vi "Main.vi"(11 "Module Admin":refnum<class "Delacor_lib_QMH_Cloneable Module Admin.lvclass">) -> ()   [LabVIEW 2024, in "ClonSubpanel.lvlib"]
doc: "This template is based off of the Queued Message Handler design pattern and the Queued Message Handler project template that ships with LabVIEW.\n\nThe main difference is that the queue is private to this module and communication between modules is performed via Broadcast and Request events.\n\nRequest events are wrapped in public API methods and are handled in the Event Handling Loop (EHL) of this VI. Any module can register for Broadcast events sent by this module. The EHL generates messages based on user interface actions.\n\nThe Message Handling Loop (MHL) processes messages generated by the EHL, or by other messages. The messages are string values, so new messages can be added easily to the Message Cases case structure in the MHL. Each message cluster can also provide an optional value for Message Data, which is a variant that can be converted to whatever message-specific data is required.\n_____\nBased on DQMH Dev Tools: Project Template 7.1.0.1503."
uses:
  ClonSubpanel.lvlib
  <vilib>/Delacor/Delacor QMH/Libraries/Cloneable Module Admin_class/Delacor_lib_QMH_Cloneable Module Admin.lvclass
  C:/Program Files (x86)/National Instruments/LabVIEW 2024/vi.lib/Delacor/Delacor QMH/Libraries/Module Admin_class/Delacor_lib_QMH_Module Admin.lvclass
  Module Data--cluster.ctl
  <vilib>/Delacor/Delacor QMH/Libraries/Message Queue_class/Delacor_lib_QMH_Message Queue.lvclass/Delacor_lib_QMH_Message Queue.ctl
  <vilib>/Delacor/Delacor QMH/Libraries/Cloneable Module Admin_class/Delacor_lib_QMH_Cloneable Module Admin.lvclass/Delacor_lib_QMH_Cloneable Module Admin.ctl
  Stop Argument--cluster.ctl
  <vilib>/Delacor/Delacor QMH/Libraries/Module Admin_class/Delacor_lib_QMH_Module Admin.lvclass/Delacor_lib_QMH_Module Admin.ctl
  Draw FP in Supbpanel Argument--cluster.ctl
  Remove FP from Subpanel Argument--cluster.ctl
  <vilib>/Utility/miscctls.llb/LVPointTypeDef.ctl
  <vilib>/Delacor/Delacor QMH/Libraries/Message Queue_class/Delacor_lib_QMH_Enqueue Message (Single).vi
  <vilib>/Delacor/Delacor QMH/Libraries/Cloneable Module Admin_class/Delacor_lib_QMH_Get Module ID.vi
  <vilib>/Delacor/Delacor QMH/Libraries/Module Admin_class/Delacor_lib_QMH_Get External Launch.vi
  <vilib>/Delacor/Delacor QMH/Libraries/Message Queue_class/Delacor_lib_QMH_Message Queue.lvclass
panel:
  out "error out":errorcluster
  out "Status":string
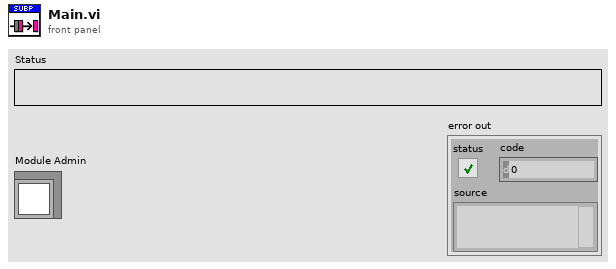
[diagram p1: front panel]
types:
  T1 = typedef "ClonSubpanel.lvlib/Request Events--cluster.ctl" = cluster{"Stop Module":refnum<user-event>, "Show Panel":refnum<user-event>, "Hide Panel":refnum<user-event>, "Show Diagram":refnum<user-event>, "Get Module Execution Status":refnum<user-event>, "Draw FP in Supbpanel":refnum<user-event>, "Remove FP from Subpanel":refnum<user-event>}
  T2 = typedef "ClonSubpanel.lvlib/Module Data--cluster.ctl" = cluster{"Status":string, "Sub Panel":refnum<vi>}
  T3 = enum32{"invalid lock state", "Not Locked", "Locked (No Password)", "Password-protected"}
  T4 = typedef "ClonSubpanel.lvlib/Stop Argument--cluster.ctl" = cluster{"Module ID":i32, "Origin":string, "Exit via Stop Module Req?":bool, "Wait for Module to stop?":bool}
  T5 = typedef "ClonSubpanel.lvlib/Draw FP in Supbpanel Argument--cluster.ctl" = cluster{"Module ID":i32, "Sub Panel":refnum<vi>}
  T6 = typedef "ClonSubpanel.lvlib/Remove FP from Subpanel Argument--cluster.ctl" = cluster{"Module ID":i32, "Boolean":bool}
  T7 = typedef "LVPointTypeDef.ctl" = cluster{"Horizontal":i16, "Vertical":i16}
  T8 = enum32{"Invalid", "Standard", "Closed", "Hidden", "Minimized", "Maximized"}
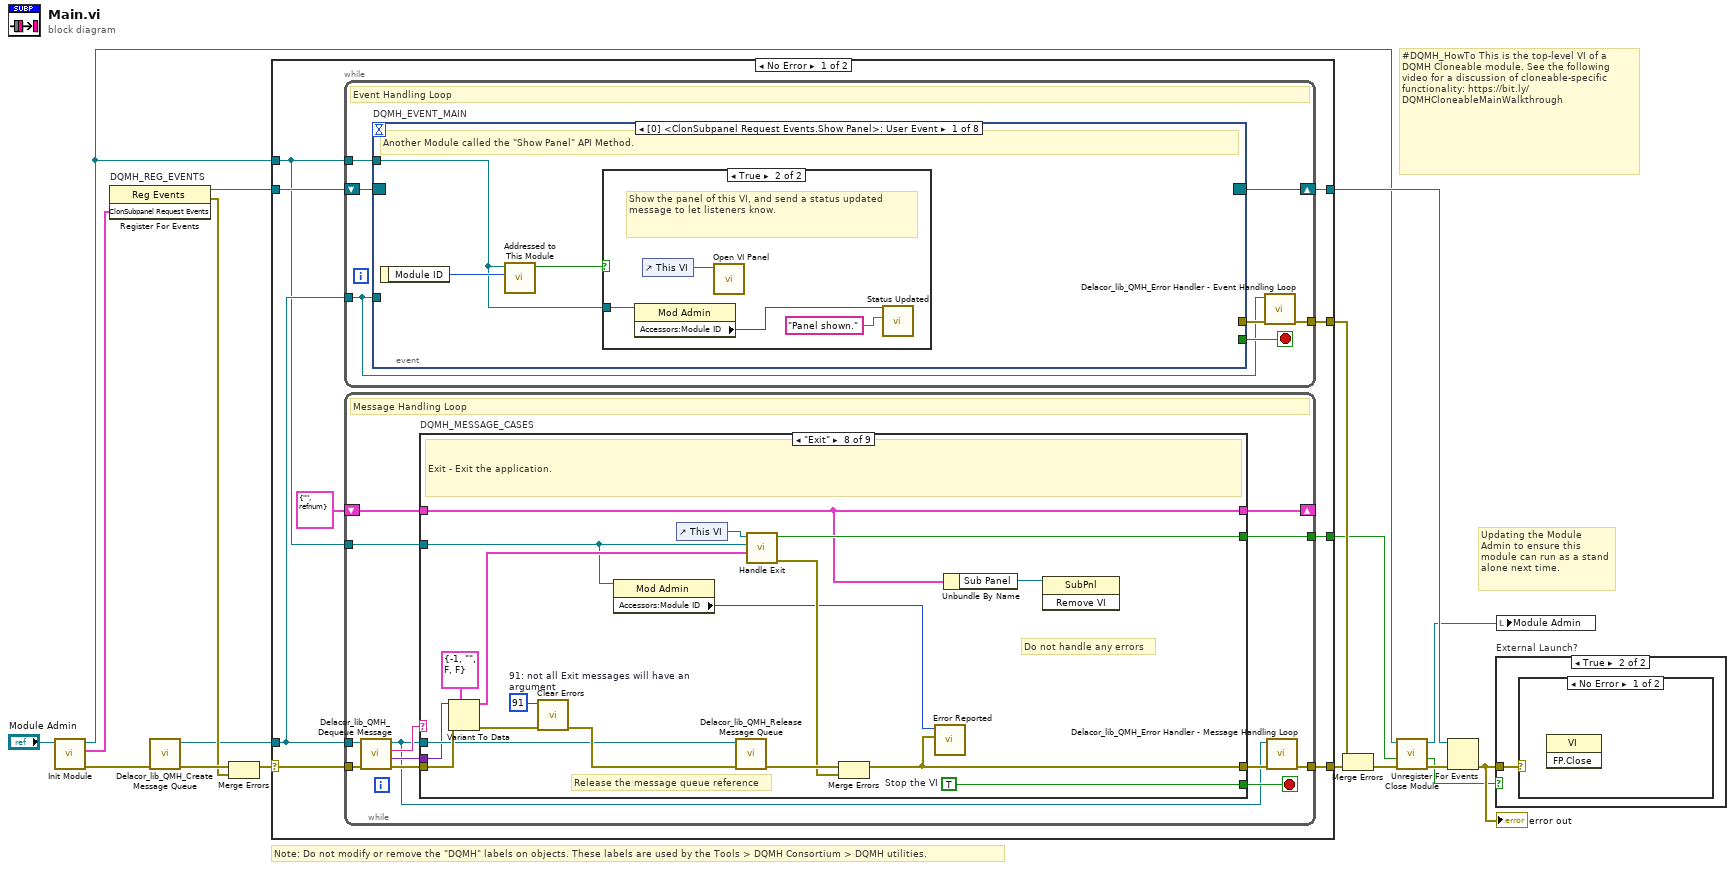
[diagram p0: block diagram]
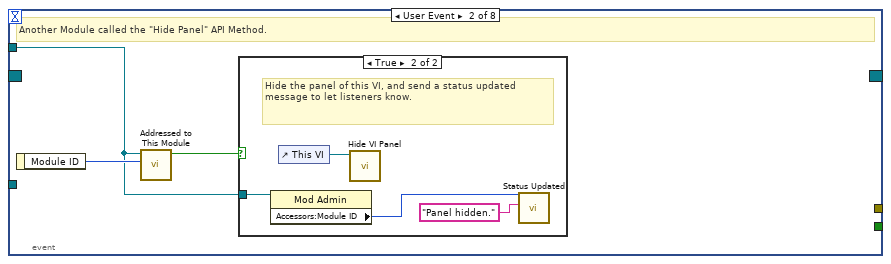
[diagram p3: hidden frame]
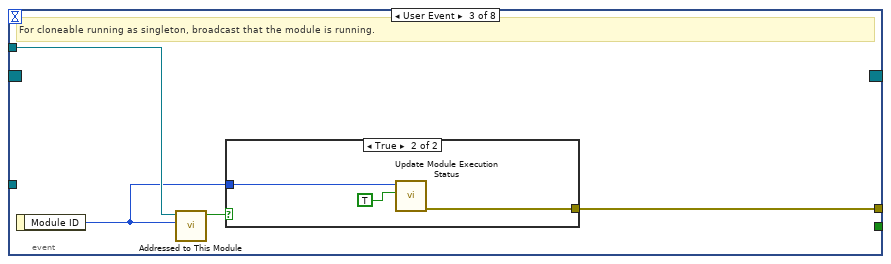
[diagram p5: hidden frame]
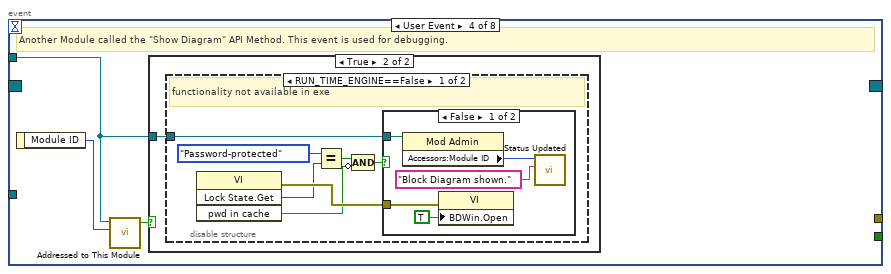
[diagram p7: hidden frame]
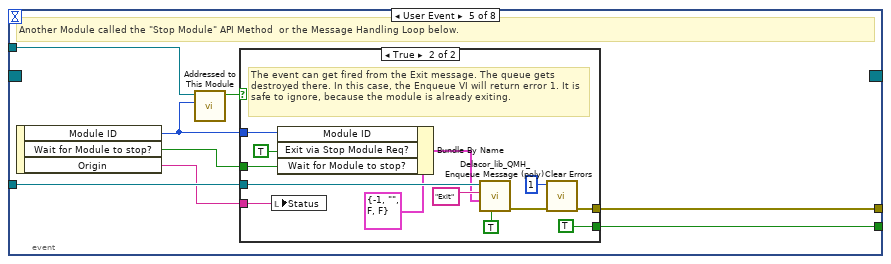
[diagram p11: hidden frame]
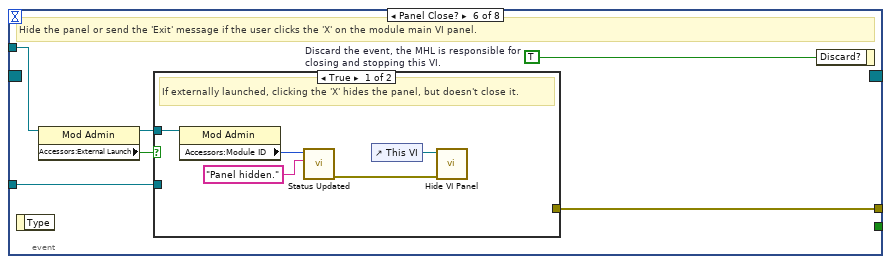
[diagram p13: hidden frame]
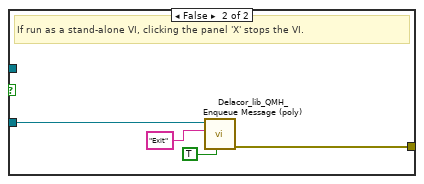
[diagram p14: hidden frame]
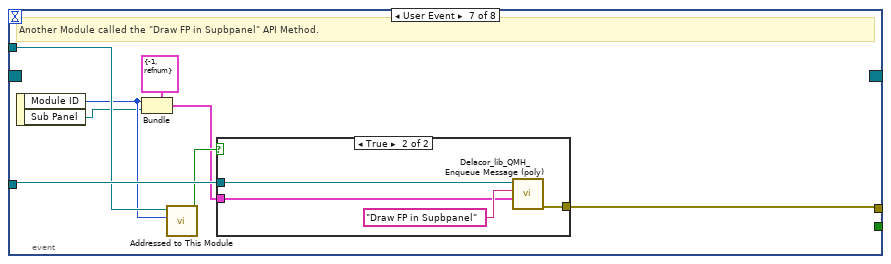
[diagram p15: hidden frame]
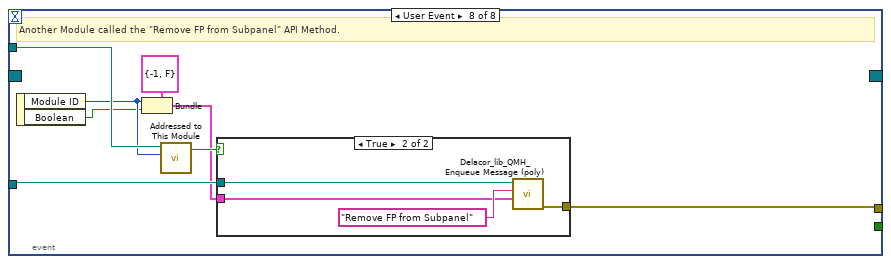
[diagram p17: hidden frame]
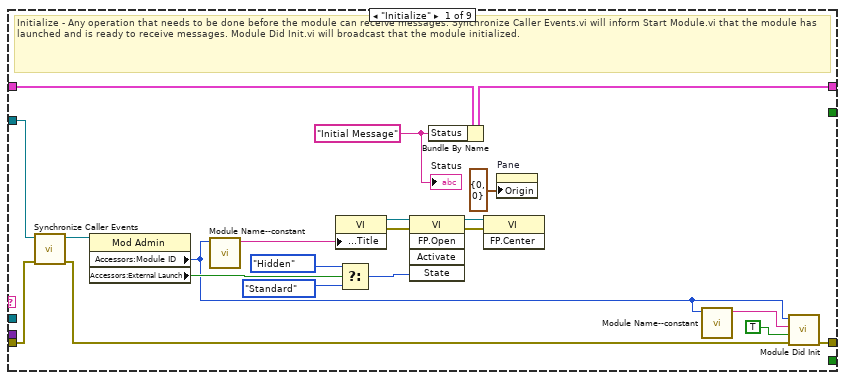
[diagram p19: hidden frame]
diagram:
  # "#DQMH_HowTo This is the top-level VI of a DQMH Cloneable module. See the following video for a discussion of cloneable-specific functionality: https://bit.ly/DQMHCloneableMainWalkthrough"
  # "Note: Do not modify or remove the \"DQMH\" labels on objects. These labels are used by the Tools > DQMH Consortium > DQMH utilities."
  # "Updating the Module Admin to ensure this module can run as a stand alone next time."
  n1 = call "Init Module.vi"("Cloneable Module Admin in"="Module Admin") -> ("error out"=w15:errorcluster, "ClonSubpanel Request Events"=w7:T1, "Cloneable Module Admin out"=w4:refnum<class "Delacor_lib_QMH_Cloneable Module Admin.lvclass">)  [unwired: 8 in]
  n2 = register-events "DQMH_REG_EVENTS"(w7) -> (reference out=w8:refnum<event-registration>, error out=w10:errorcluster)  [unwired: 2 in]
  n3 = call <vilib>:"Delacor_lib_QMH_Create Message Queue.vi"("error in"=w15) -> ("error out"=w12:errorcluster, "Message Queue"=w6:refnum<class "Delacor_lib_QMH_Message Queue.lvclass">)  [unwired: 9 in]
  n4 = Merge Errors(w12, w10) -> (w11:errorcluster)
  n5 = case shown="No Error" w11 {
    selector: w11 -> [w25 w267]
    tunnel: [w27 w266] -> w16
    tunnel: [w24 w265] -> w9
    tunnel: w8 -> [w22 w265]
    tunnel: w6 -> [w21 w258]
    tunnel: [w26 _] -> w17
    tunnel: w4 -> [w20 w261]
    tunnel: [w19 _] -> w2
    frame No Error {
      n6 = while {
        tunnel: w21 -> [w28]
        shift-right: [w31] -> w24
        shift-left: w22 -> [w32]
        tunnel: [w33] -> w26
        tunnel: w20 -> [w29]
        stop <- w30 stop-if-true
        # "Event Handling Loop"
        n7 = event "DQMH_EVENT_MAIN" shown="[0] <ClonSubpanel Request Events.Show Panel>: User Event" {
          selector: w32 -> [_ _ _ _ _ _ _ _]
          dyn-events: [_ _ _ _ _ _ _ _] -> w31
          timeout: _ -> [_ _ _ _ _ _ _ _]
          tunnel: [_ _ _ _ w75 _ _ _] -> w30
          tunnel: w28 -> [_ _ _ _ w78 w95 w115 w127]
          tunnel: [_ _ w52 _ w79 w98 w108 w120] -> w34
          tunnel: w29 -> [w35 w42 w50 w56 w77 w96 w113 w125]
          event User Event {
            # "Another Module called the \"Show Panel\" API Method."
            n8 = event-data() -> ("Module ID"=w36:i32)  [unwired: 1 in]
            n9 = call "Addressed to This Module.vi"("Module ID from Argument"=w36, "Module Admin"=w35) -> ("Addressed to this instance?"=w37:bool)  [unwired: 8 in, 1 out]
            n10 = case shown="True" w37 {
              tunnel: w35 -> [_ w39]
              frame False {
              }
              frame True {
                # "Show the panel of this VI, and send a status updated message to let listeners know."
                n11 = property on="Property Node" class="Mod Admin"(reference=w39) -> ("Accessors:Module ID"=w38:i32)  [unwired: 1 in, 2 out]
                n12 = control-ref of="This VI"() -> (w41:refnum<vi>)
                n13 = call "Open VI Panel.vi"("VI"=w41) -> ()  [unwired: 10 in, 1 out]
                n14 = call "Status Updated.vi"("Status"="Panel shown." ("format string"), "Module ID"=w38) -> ()  [unwired: 9 in, 1 out]
              }
            }
          }
          event User Event {
            # "Another Module called the \"Hide Panel\" API Method."
            n15 = event-data() -> ("Module ID"=w43:i32)  [unwired: 1 in]
            n16 = call "Addressed to This Module.vi"("Module ID from Argument"=w43, "Module Admin"=w42) -> ("Addressed to this instance?"=w44:bool)  [unwired: 8 in, 1 out]
            n17 = case shown="True" w44 {
              tunnel: w42 -> [_ w46]
              frame False {
              }
              frame True {
                # "Hide the panel of this VI, and send a status updated message to let listeners know."
                n18 = property on="Property Node" class="Mod Admin"(reference=w46) -> ("Accessors:Module ID"=w45:i32)  [unwired: 1 in, 2 out]
                n19 = control-ref of="This VI"() -> (w48:refnum<vi>)
                n20 = call "Hide VI Panel.vi"("VI"=w48) -> ()  [unwired: 10 in, 1 out]
                n21 = call "Status Updated.vi"("Status"="Panel hidden." ("format string"), "Module ID"=w45) -> ()  [unwired: 9 in, 1 out]
              }
            }
          }
          event User Event {
            # "For cloneable running as singleton, broadcast that the module is running."
            n22 = event-data() -> ("Module ID"=w49:i32)  [unwired: 1 in]
            n23 = call "Addressed to This Module.vi"("Module ID from Argument"=w49, "Module Admin"=w50) -> ("Addressed to this instance?"=w51:bool)  [unwired: 8 in, 1 out]
            n24 = case shown="True" w51 {
              tunnel: [_ w55] -> w52
              tunnel: w49 -> [_ w54]
              frame False {
              }
              frame True {
                n25 = call "Update Module Execution Status.vi"("Running?"=TRUE, "Module ID"=w54) -> ("error out"=w55:errorcluster)  [unwired: 9 in]
              }
            }
          }
          event User Event {
            # "Another Module called the \"Show Diagram\" API Method. This event is used for debugging."
            n26 = event-data() -> ("Module ID"=w57:i32)  [unwired: 1 in]
            n27 = call "Addressed to This Module.vi"("Module ID from Argument"=w57, "Module Admin"=w56) -> ("Addressed to this instance?"=w58:bool)  [unwired: 8 in, 1 out]
            n28 = case shown="True" w58 {
              tunnel: w56 -> [_ w59]
              frame False {
              }
              frame True {
                n29 = disable-structure shown="RUN_TIME_ENGINE==False" {
                  disable-tunnel: w59 -> [w60 _]
                  frame condition #0 (active) {
                    # "functionality not available in exe"
                    n30 = invoke on="Invoke Node" class="VI" method="Lock State.Get"() -> (error out=w66:errorcluster, "Get Lock State"=w65:T3, "pwd in cache"=w62:bool)  [unwired: 4 in, 1 out]
                    n31 = Equal?(x=T3."Password-protected", y=w65) -> (x = y?=w63:bool)
                    n32 = Compound Arithmetic op=AND(w63, invert w62) -> (w61:bool)
                    n33 = case shown="False" w61 {
                      tunnel: w66 -> [w71 _]
                      tunnel: w60 -> [w68 _]
                      frame False {
                        n34 = property on="Property Node" class="Mod Admin"(reference=w68) -> ("Accessors:Module ID"=w67:i32)  [unwired: 1 in, 2 out]
                        n35 = property on="Property Node" class="VI"(error in=w71, "BDWin.Open"=TRUE ("Block Diagram Window:Open")) -> ()  [unwired: 1 in, 2 out]
                        n36 = call "Status Updated.vi"("Status"="Block Diagram shown." ("format string"), "Module ID"=w67) -> ()  [unwired: 9 in, 1 out]
                      }
                      frame True {
                        # "Password-protected VI, and the password is not in the cache. Do not show the diagram."
                      }
                    }
                  }
                  frame condition #1 {
                  }
                }
              }
            }
          }
          event User Event {
            # "Another Module called the \"Stop Module\" API Method  or the Message Handling Loop below."
            n37 = event-data() -> ("Module ID"=w73:i32, "Wait for Module to stop?"=w74:bool, "Origin"=w72:string)  [unwired: 1 in]
            n38 = call "Addressed to This Module.vi"("Module ID from Argument"=w73, "Module Admin"=w77) -> ("Addressed to this instance?"=w76:bool)  [unwired: 8 in, 1 out]
            n39 = case shown="True" w76 {
              tunnel: [_ w91] -> w79
              tunnel: w78 -> [_ w87]
              tunnel: [_ TRUE] -> w75
              tunnel: w74 -> [_ w82]
              tunnel: w73 -> [_ w84]
              tunnel: w72 -> [_ w80]
              frame False {
              }
              frame True {
                # "The event can get fired from the Exit message. The queue gets destroyed there. In this case, the Enqueue VI will return error 1. It is safe to ignore, because the module is already exiting."
                n40 = local write "Status"(w80) -> ()
                n41 = Bundle By Name(cluster=T4 {"Module ID"=-1, "Origin"="", "Exit via Stop Module Req?"=FALSE, "Wait for Module to stop?"=FALSE} ("Stop Argument"), "Module ID"=w84, "Exit via Stop Module Req?"=TRUE, "Wait for Module to stop?"=w82) -> (w81:T4)
                n42 = call-poly <vilib>:"Delacor_lib_QMH_Enqueue Message (poly).vi"("Priority Message? (F)"=TRUE, "Message Data"=w81, "Message"="Exit", "Message Queue in"=w87) -> ("error out"=w92:errorcluster)  [unwired: 6 in, 1 out]
                n43 = call <vilib>:"Clear Errors.vi"("error in (no error)"=w92, "specific error code to clear (0: all)"=1) -> ("error out"=w91:errorcluster)  [unwired: 4 in, 1 out]
              }
            }
          }
          event Panel Close? {
            w97 = TRUE  # Discard the event, the MHL is responsible for closing and stopping this VI.
            # "Hide the panel or send the 'Exit' message if the user clicks the 'X' on the module main VI panel."
            n44 = event-data() -> ()  [unwired: 1 in, 1 out]
            n45 = property on="Property Node" class="Mod Admin"(reference=w96) -> (reference out=w93:refnum<class "Delacor_lib_QMH_Cloneable Module Admin.lvclass">, "Accessors:External Launch"=w94:bool)  [unwired: 1 in, 1 out]
            n46 = case shown="True" w94 {
              tunnel: w95 -> [_ w106]
              tunnel: [_ w107] -> w98
              tunnel: w93 -> [w101 _]
              frame True {
                # "If externally launched, clicking the 'X' hides the panel, but doesn't close it."
                n47 = property on="Property Node" class="Mod Admin"(reference=w101) -> ("Accessors:Module ID"=w100:i32)  [unwired: 1 in, 2 out]
                n48 = call "Status Updated.vi"("Status"="Panel hidden." ("format string"), "Module ID"=w100) -> ("error out"=w99:errorcluster)  [unwired: 9 in]
                n49 = control-ref of="This VI"() -> (w103:refnum<vi>)
                n50 = call "Hide VI Panel.vi"("error in"=w99, "VI"=w103) -> ()  [unwired: 9 in, 1 out]
              }
              frame False {
                # "If run as a stand-alone VI, clicking the panel 'X' stops the VI."
                n51 = call-poly <vilib>:"Delacor_lib_QMH_Enqueue Message (poly).vi"("Priority Message? (F)"=TRUE, "Message"="Exit", "Message Queue in"=w106) -> ("error out"=w107:errorcluster)  [unwired: 7 in, 1 out]
              }
            }
            n52 = event-data ("Event Filter Node")("Discard?"=w97) -> ()  [unwired: 1 in, 1 out]
          }
          event User Event {
            # "Another Module called the \"Draw FP in Supbpanel\" API Method."
            n53 = event-data() -> ("Module ID"=w110:i32, "Sub Panel"=w109:refnum<vi>)  [unwired: 1 in]
            n54 = Bundle(cluster=T5 {"Module ID"=-1, "Sub Panel"=refnum} ("Draw FP in Supbpanel Argument"), "Module ID"=w110, "Sub Panel"=w109) -> (w111:T5)
            n55 = call "Addressed to This Module.vi"("Module ID from Argument"=w110, "Module Admin"=w113) -> ("Addressed to this instance?"=w114:bool)  [unwired: 8 in, 1 out]
            n56 = case shown="True" w114 {
              tunnel: w115 -> [_ w119]
              tunnel: w111 -> [_ w117]
              tunnel: [_ w116] -> w108
              frame False {
              }
              frame True {
                n57 = call-poly <vilib>:"Delacor_lib_QMH_Enqueue Message (poly).vi"("Message Data"=w117, "Message"="Draw FP in Supbpanel", "Message Queue in"=w119) -> ("error out"=w116:errorcluster)  [unwired: 7 in, 1 out]
              }
            }
          }
          event User Event {
            # "Another Module called the \"Remove FP from Subpanel\" API Method."
            n58 = event-data() -> ("Module ID"=w122:i32, "Boolean"=w121:bool)  [unwired: 1 in]
            n59 = Bundle(cluster=T6 {"Module ID"=-1, "Boolean"=FALSE} ("Remove FP from Subpanel Argument"), "Module ID"=w122, "Boolean"=w121) -> (w123:T6)
            n60 = call "Addressed to This Module.vi"("Module ID from Argument"=w122, "Module Admin"=w125) -> ("Addressed to this instance?"=w126:bool)  [unwired: 8 in, 1 out]
            n61 = case shown="True" w126 {
              tunnel: w127 -> [_ w131]
              tunnel: w123 -> [_ w129]
              tunnel: [_ w128] -> w120
              frame False {
              }
              frame True {
                n62 = call-poly <vilib>:"Delacor_lib_QMH_Enqueue Message (poly).vi"("Message Data"=w129, "Message"="Remove FP from Subpanel", "Message Queue in"=w131) -> ("error out"=w128:errorcluster)  [unwired: 7 in, 1 out]
              }
            }
          }
        }
        n63 = call-dynamic "Delacor_lib_QMH_Error Handler - Event Handling Loop.vi"("error in"=w34, "Message Queue in"=w28) -> ("dup error in"=w33:errorcluster)  [unwired: 8 in, 1 out]
      }
      n64 = while {
        tunnel: w21 -> [w132]
        shift-right: [w139] -> _
        shift-left: T2 {"Status"="", "Sub Panel"=refnum} ("Data Cluster") -> [w140]
        tunnel: w25 -> [w143]
        tunnel: [w141] -> w27
        tunnel: w20 -> [w134]
        tunnel: [w133] -> w19
        stop <- w138 stop-if-true
        # "Message Handling Loop"
        n65 = call-dynamic "Delacor_lib_QMH_Dequeue Message.vi"("error in"=w143, "Message Queue in"=w132) -> ("error out"=w142:errorcluster, "Message Data"=w136:variant, "Message"=w137:string, "Message Queue out"=w135:refnum<class "Delacor_lib_QMH_Message Queue.lvclass">)  [unwired: 6 in]
        n66 = case "DQMH_MESSAGE_CASES" shown="\"Exit\"" w137 {
          selector: w137 -> [_ _ _ _ _ _ _ _ w247]
          tunnel: w135 -> [_ _ _ _ _ _ w212 w239 _]
          tunnel: w142 -> [w163 w167 w183 w200 w207 w209 w221 w245 w256]
          tunnel: [w161 w167 w177 w194 w206 w209 w217 w240 w257] -> w144
          tunnel: w140 -> [w154 w166 w182 w196 w205 w208 w216 w229 w254]
          tunnel: [w153 w166 w169 w191 w205 w208 w216 w229 w254] -> w139
          tunnel: [_ _ _ _ _ _ _ w238 _] -> w138
          tunnel: w136 -> [_ _ w180 w199 _ _ w215 w236 _]
          tunnel: w134 -> [w149 _ _ _ _ _ w214 w231 w253]
          tunnel: [_ _ _ _ _ _ _ w234 _] -> w133
          frame "Initialize" {
            w146 = "Initial Message" ("Initial Message")
            # "Initialize - Any operation that needs to be done before the module can receive messages. Synchronize Caller Events.vi will inform Start Module.vi that the module has launched and is ready to receive messages. Module Did Init.vi will broadcast that the module initialized."
            n67 = call "Synchronize Caller Events.vi"("error in"=w163, "Module Admin"=w149) -> ("error out"=w162:errorcluster, "Module Admin out"=w148:refnum<class "Delacor_lib_QMH_Cloneable Module Admin.lvclass">)  [unwired: 8 in]
            n68 = property on="Property Node" class="Mod Admin"(reference=w148) -> ("Accessors:Module ID"=w145:i32, "Accessors:External Launch"=w150:bool)  [unwired: 1 in, 2 out]
            n69 = call "Module Name--constant.vi"("Module ID"=w145) -> ("Module Name"=w158:string)  [unwired: 10 in]
            n70 = property on="Property Node" class="VI"("Front Panel.Title"=w158) -> (reference out=w160:refnum<vi>, error out=w165:errorcluster)  [unwired: 2 in]
            n71 = Select(t=T8."Hidden" ("State"), s=w150, f=T8."Standard" ("State")) -> (s? t:f=w155:T8)
            n72 = invoke on="Invoke Node" class="VI" method="FP.Open"(reference=w160, error in=w165, "State"=w155) -> (reference out=w159:refnum<vi>, error out=w164:errorcluster)  [unwired: 2 in, 3 out]
            n73 = Bundle By Name(cluster=w154, "Status"=w146) -> (w153:T2)
            n74 = invoke on="Invoke Node" class="VI" method="FP.Center"(reference=w159, error in=w164) -> ()  [unwired: 1 in, 3 out]
            n75 = property on="Pane" class="Pane"("Origin"=T7 {"Horizontal"=0, "Vertical"=0}) -> ()  [unwired: 2 in, 2 out]
            n76 = call "Module Name--constant.vi"("Module ID"=w145) -> ("Module Name"=w151:string)  [unwired: 10 in]
            n77 = call "Module Did Init.vi"("error in"=w162, "Initialized?"=TRUE, "Origin"=w151, "Module ID"=w145) -> ("error out"=w161:errorcluster)  [unwired: 7 in]
            "Status" <- w146
          }
          frame "---Module Specific---" {
            # "Separator -- The following cases handle messages specific to this Module."
          }
          frame "Draw FP in Supbpanel" {
            # "Draw FP in Supbpanel"
            n78 = Variant To Data(error in=w183, type=T5 {"Module ID"=-1, "Sub Panel"=refnum} ("Draw FP in Supbpanel Argument"), Variant=w180) -> (data=w178:T5, error out=w181:errorcluster)
            n79 = Unbundle By Name(w178) -> ("Sub Panel"=w176:refnum<vi>)
            n80 = control-ref of="This VI"() -> (w175:refnum<vi>)
            n81 = property class="VI"(reference=w175, error in=w181) -> (reference out=w173:refnum<vi>, error out=w172:errorcluster, "FP.State"=w174:T8)
            n82 = case shown="Default" w174 {
              tunnel: w173 -> [w187 w189]
              tunnel: w172 -> [w186 w188]
              tunnel: [w185 w188] -> w170
              tunnel: [w184 w189] -> w171
              frame Default {
                n83 = invoke class="VI" method="FP.Close"(reference=w187, error in=w186) -> (reference out=w184:refnum<vi>, error out=w185:errorcluster)  [unwired: 1 in, 1 out]
              }
              frame "Closed" {
              }
            }
            n84 = invoke class="SubPnl" method="Insert VI"(reference=w176, error in=w170, "VI Ref"=w171) -> (reference out=w168:refnum<vi>, error out=w177:errorcluster)  [unwired: 1 in, 2 out]
            n85 = Bundle By Name(cluster=w182, "Sub Panel"=w168) -> (w169:T2)
          }
          frame "Remove FP from Subpanel" {
            # "Remove FP from Subpanel"
            n86 = Variant To Data(error in=w200, type=T6 {"Module ID"=-1, "Boolean"=FALSE} ("Remove FP from Subpanel Argument"), Variant=w199) -> (data=w197:T6, error out=w195:errorcluster)
            n87 = Unbundle By Name(w197) -> ()  [unwired: 2 out]
            n88 = Unbundle By Name(w196) -> ("Sub Panel"=w193:refnum<vi>)
            n89 = Not A Number/Path/Refnum?(number/path/refnum=w193) -> (NaN/Path/Refnum?=w192:bool)
            n90 = case shown="False" w192 {
              tunnel: w195 -> [w203 w204]
              tunnel: [w202 w204] -> w194
              tunnel: w193 -> [w201 _]
              frame False {
                n91 = invoke class="SubPnl" method="Remove VI"(reference=w201, error in=w203) -> (error out=w202:errorcluster)  [unwired: 1 in, 2 out]
              }
              frame True {
              }
            }
            n92 = Bundle By Name(cluster=w196, "Sub Panel"=refnum<vi> refnum) -> (w191:T2)
          }
          frame "---Copy This Frame---" {
            # "Duplicate this frame when creating new messages.  Change this comment in the duplicated frame to describe this message."
            n93 = Merge Errors(w207) -> (w206:errorcluster)
          }
          frame "---Exit and Error Handling---" {
            # "Separator - the following cases handle errors and exit messages."
          }
          frame "Error" {
            # "#DQMH_CodeRecommended - If the module is running in standalone mode (External Launch = FALSE), this code will pop up an error dialog and call the 'Exit' message if an error occurs. Add more fine-grained error management here."
            # "Error - Check the error message data and respond accordingly. This message is sent by the \"Error Handler\" VIs at the end of each loop in this application."
            n94 = property on="Property Node" class="Mod Admin"(reference=w214) -> ("Accessors:External Launch"=w213:bool, "Accessors:Module ID"=w211:i32)  [unwired: 1 in, 2 out]
            n95 = Variant To Data(error in=w221, type=errorcluster {"status"=FALSE, "code"=0, "source"=""} ("error constant"), Variant=w215) -> (data=w210:errorcluster, error out=w219:errorcluster)
            n96 = local write "error out"(w210) -> ()
            n97 = call "Error Reported.vi"("Error"=w210, "Module ID"=w211) -> ()  [unwired: 9 in, 1 out]
            n98 = case shown="False" w213 {
              tunnel: [w226 _] -> w218
              tunnel: w212 -> [w224 _]
              tunnel: w210 -> [w225 _]
              frame False {
                n99 = disable-structure shown="Default" {
                  disable-tunnel: w225 -> [w227 _]
                  frame condition #0 (active) {
                    # "If the module is running standalone, then pop up an error dialog and call the \"Exit\" message."
                    n100 = call <vilib>:"Simple Error Handler.vi"("error in (no error)"=w227) -> ()  [unwired: 4 in, 5 out]
                  }
                  frame condition #1 {
                    # "To prevent the Simple Error Handler VI from being loaded (e.g. when deploying to a Real-Time target), add the Conditional Disable Symbol \"DQMH_Disable_SEH\" to your project and set it to TRUE."
                  }
                }
                n101 = call-poly <vilib>:"Delacor_lib_QMH_Enqueue Message (poly).vi"("Priority Message? (F)"=TRUE, "Message"="Exit", "Message Queue in"=w224) -> ("error out"=w226:errorcluster)  [unwired: 7 in, 1 out]
              }
              frame True {
                # "If the module was launched externally, calling the Error Reported broadcast VI is the only action performed by the \"Error\" message. The module's caller can then process the error appropriately."
              }
            }
            n102 = Merge Errors(w219, w218) -> (w217:errorcluster)
          }
          frame "Exit" {
            w237 = 91  # 91: not all Exit messages will have an argument
            w238 = TRUE  # Stop the VI
            # "Do not handle any errors"
            # "Release the message queue reference"
            # "Exit - Exit the application."
            n103 = Variant To Data(error in=w245, type=T4 {"Module ID"=-1, "Origin"="", "Exit via Stop Module Req?"=FALSE, "Wait for Module to stop?"=FALSE} ("Stop Argument"), Variant=w236) -> (data=w233:T4, error out=w241:errorcluster)
            n104 = call <vilib>:"Clear Errors.vi"("error in (no error)"=w241, "specific error code to clear (0: all)"=w237) -> ("error out"=w244:errorcluster)  [unwired: 4 in, 1 out]
            n105 = property on="Property Node" class="Mod Admin"(reference=w231) -> ("Accessors:Module ID"=w230:i32)  [unwired: 1 in, 2 out]
            n106 = control-ref of="This VI"() -> (w232:refnum<vi>)
            n107 = call-dynamic "Delacor_lib_QMH_Release Message Queue.vi"("error in"=w244, "Message Queue"=w239) -> ("error out"=w243:errorcluster)  [unwired: 9 in]
            n108 = call "Handle Exit.vi"("Stop Argument"=w233, "Module Admin in"=w231, "VI reference"=w232) -> ("error out"=w242:errorcluster, "Wait for Stop?"=w234:bool)  [unwired: 7 in]
            n109 = Merge Errors(w243, w242) -> (w240:errorcluster)
            n110 = call "Error Reported.vi"("Error"=w240, "Module ID"=w230) -> ()  [unwired: 9 in, 1 out]
            n111 = Unbundle By Name(w229) -> ("Sub Panel"=w228:refnum<vi>)
            n112 = invoke class="SubPnl" method="Remove VI"(reference=w228) -> ()  [unwired: 2 in, 3 out]
          }
          frame Default {
            # "'Default' case only runs if there is a message that isn't defined in any of the other cases.  Output a programming error."
            n113 = property on="Property Node" class="Mod Admin"(reference=w253) -> ("Accessors:Module ID"=w252:i32)  [unwired: 1 in, 2 out]
            n114 = call "Module Name--constant.vi"("Module ID"=w252) -> ("Module Name"=w246:string)  [unwired: 10 in]
            n115 = Format Into String(format string="The invalid message string \"%s\" was received in the Message Handling Loop for module \"%s\".", w247, w246) -> (resulting string=w249:string)  [unwired: 2 in, 1 out]
            n116 = call <vilib>:"Error Cluster From Error Code.vi"("show call chain? (False)"=TRUE, "error message (\"\")"=w249, "error code (0)"=1) -> ("error out"=w255:errorcluster)  [unwired: 6 in]
            n117 = Merge Errors(w256, w255) -> (w257:errorcluster)
          }
        }
        n118 = call-dynamic "Delacor_lib_QMH_Error Handler - Message Handling Loop.vi"("error in"=w144, "Message Queue in"=w135) -> ("dup error in"=w141:errorcluster)  [unwired: 8 in, 1 out]
      }
    }
    frame Error {
      n119 = call "Synchronize Caller Events.vi"("Module Admin"=w261) -> ("Module Admin out"=w260:refnum<class "Delacor_lib_QMH_Cloneable Module Admin.lvclass">)  [unwired: 9 in, 1 out]
      n120 = property on="Property Node" class="Mod Admin"(reference=w260) -> ("Accessors:Module ID"=w259:i32)  [unwired: 1 in, 2 out]
      n121 = call-dynamic "Delacor_lib_QMH_Release Message Queue.vi"("error in"=w267, "Message Queue"=w258) -> ("error out"=w266:errorcluster)  [unwired: 9 in]
      n122 = call "Module Name--constant.vi"("Module ID"=w259) -> ("Module Name"=w264:string)  [unwired: 10 in]
      n123 = Format Into String(format string="An error occurred during initialization. %s is no longer running.", w264) -> (resulting string=w262:string)  [unwired: 2 in, 1 out]
      n124 = call "Error Reported.vi"("Additional Information"=w262, "Error"=w266, "Module ID"=w259) -> ()  [unwired: 8 in, 1 out]
    }
  }
  n125 = Merge Errors(w17, w16) -> (w18:errorcluster)
  n126 = call "Close Module.vi"("error in"=w18, "Wait for stop?"=w2, "Module Admin in"=w4) -> ("error out"=w14:errorcluster, "External Launch"=w1:bool, "Module Admin out"=w3:refnum<class "Delacor_lib_QMH_Cloneable Module Admin.lvclass">)  [unwired: 6 in]
  n127 = Unregister For Events(event registration refnum=w9, error in=w14) -> (error out=w13:errorcluster)
  "error out" <- w13
  n128 = case "External Launch?" shown="True" w1 {
    tunnel: w13 -> [_ w268]
    frame False {
    }
    frame True {
      n129 = case shown="No Error" w268 {
        frame No Error {
          n130 = invoke class="VI" method="FP.Close"() -> ()  [unwired: 3 in, 3 out]
        }
        frame Error {
          n131 = disable-structure shown="Default" {
            frame condition #0 (active) {
              n132 = invoke class="VI" method="FP.Open"("Activate"=TRUE ("Activate?")) -> ()  [unwired: 4 in, 5 out]
            }
            frame condition #1 {
              # "Don't show panel on error if running inside a built EXE."
            }
          }
        }
      }
    }
  }
  n133 = local write "Module Admin"(w3) -> ()
